vi "Set_Prompt.vi"(1 "Prompt":string, 2 "Argument List In":string[](array[string])) -> (0 "Argument List Out":string[](array[string]))   [LabVIEW 2011]
doc: "This VI sets a prompt to be displayed to the user for an API function that is required to wait for user input."
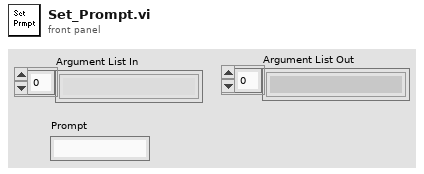
[diagram p1: front panel]
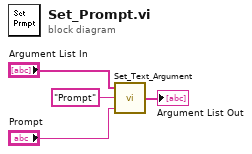
[diagram p0: block diagram]
diagram:
  n1 = call "Set_Text_Argument.vi"("Text"="Prompt", "Argument"="Prompt", "Argument List In"="Argument List In") -> ("Argument List Out"=→"Argument List Out":string[])
